vi "Test4.vi"() -> ()   [LabVIEW 2017]
panel:
  in  "String":string
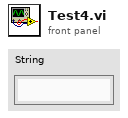
[diagram p1: front panel]
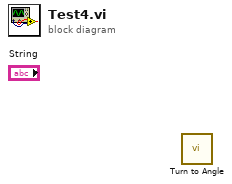
[diagram p0: block diagram]
diagram:
  n1 = call "Turn to Angle.vi"() -> ()  [unwired: 15 in, 1 out]
